vi "UserInput.vi"(1 "prompt":string) -> (0 "user input":string)   [LabVIEW 2014, in "Raspberry Pi Compatible Compiler for LabVIEW.lvlib" / "Console.lvlib"]
doc: "Prompts a user for input from stdin. The optional prompt parameter provides a prompt message without requiring a separate print command."
uses:
  Console.lvlib
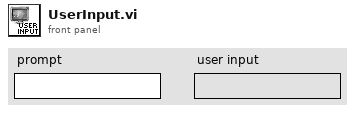
[diagram p1: front panel]
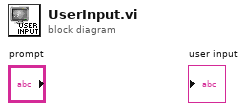
[diagram p0: block diagram]
diagram:
